vi "testArangeIdx.vi"(8 "error in (no error)":errorcluster) -> (0 "error out":errorcluster)   [LabVIEW 2016]
doc: "Test to generate the index array."
uses:
  <vilib>/addons/_JKI Toolkits/Caraya/classes/Assert/Assert.lvclass
  <vilib>/addons/_JKI Toolkits/Caraya/classes/Test/Test.lvclass
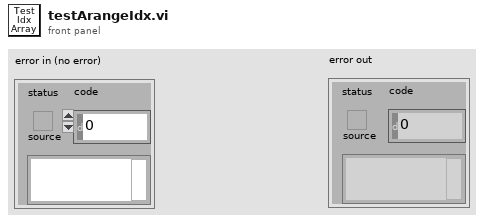
[diagram p1: front panel]
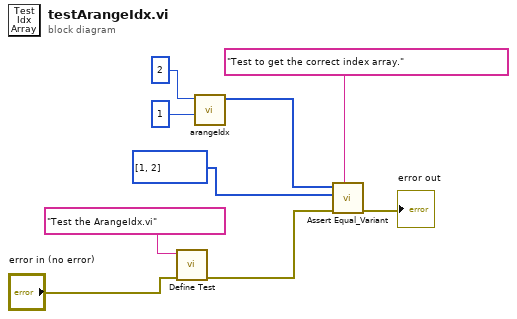
[diagram p0: block diagram]
diagram:
  n1 = call <vilib>:"Define Test.vi"("error in (no error)"="error in (no error)", "Label (VI Title)"="Test the ArangeIdx.vi") -> ("error out"=w2:errorcluster)  [unwired: 9 in]
  n2 = call "arangeIdx.vi"("Offset"=1, "Number"=2) -> ("Idx Array"=w5:i32[])  [unwired: 9 in]
  n3 = call <vilib>:"Assert Equal_Variant.vi"("Label"="Test to get the correct index array.", "error in (no error)"=w2, "Y"=i32[] [1, 2], "X"=w5) -> ("error out"=→"error out":errorcluster)  [unwired: 7 in]
